vi "故障告警分析.vi"(8 "告警代码":u16, 9 "故障代码":u16, 10 "运行步序":u16, 11 "参数":string) -> (1 "报警簇":T1, 2 "报警内容":T2, 3 "简易报警状态":cluster{"故障状态":string, "报警状态":string}, 5 "sysid":i32)   [LabVIEW 2016, in "斯坦道氨氮.lvlib"]
panel:
  in  "氨氮报警":string[][](array[string])
  # "1、注射泵水样阀口堵塞；\n2、注射泵阀过载或丝杆无动作。"
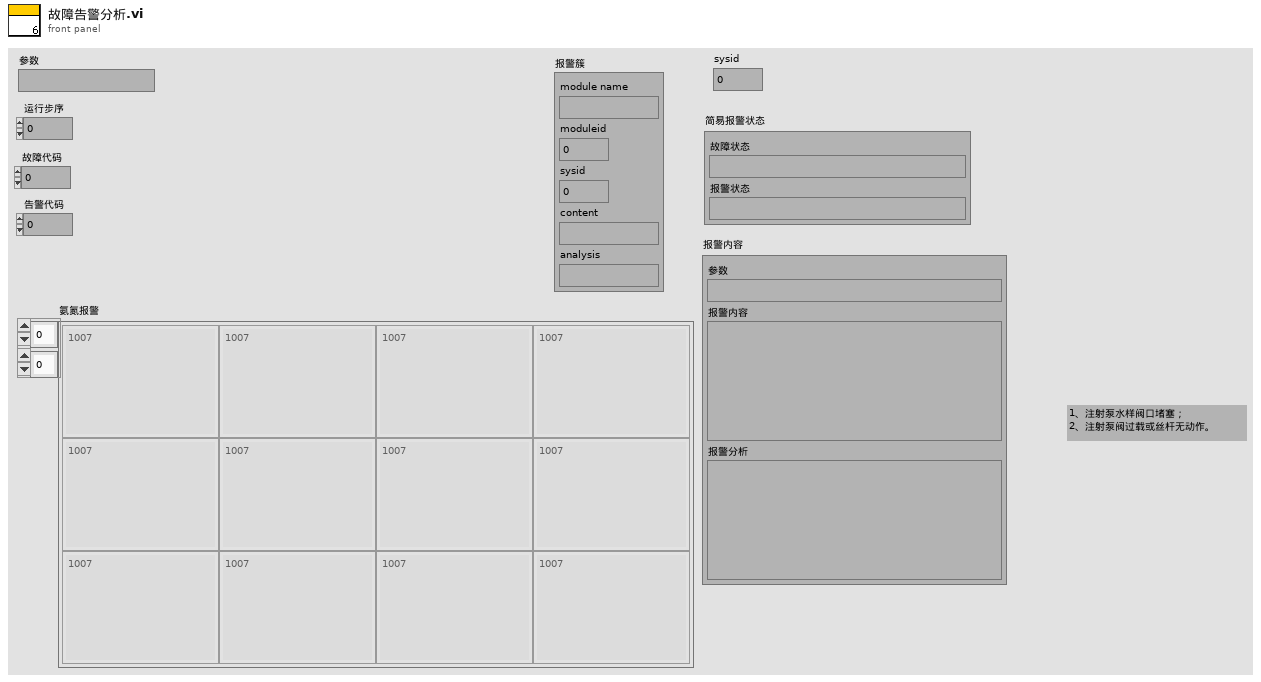
[diagram p1: front panel]
types:
  T1 = cluster{"module name":string, "moduleid":i32, "sysid":i32, "content":string, "analysis":string}
  T2 = cluster{"参数":string, "报警内容":string, "报警分析":string}
  T3 = cluster{"modid":i32, "sysid":i32, "content":string, "故障详情":string}
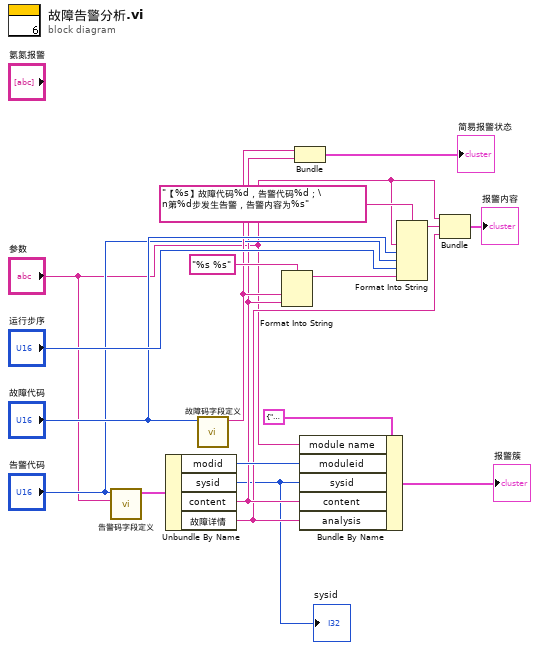
[diagram p0: block diagram]
diagram:
  n1 = call "告警码字段定义.vi"("模块名称"="参数", "告警代码"="告警代码") -> ("报警"=w6:T3)  [unwired: 9 in]
  n2 = Unbundle By Name(w6) -> ("modid"=w5:i32, "sysid"=w1:i32, "content"=w4:string, "故障详情"=w3:string)
  "sysid" <- w1
  n3 = call "故障码字段定义.vi"("故障代码"="故障代码") -> ("字符串"=w12:string)  [unwired: 10 in]
  n4 = Format Into String(format string="%s %s" ("格式字符串"), w12, w4) -> (resulting string=w8:string)  [unwired: 2 in, 1 out]
  n5 = Bundle("字符串"=w12, "content"=w4) -> (→"简易报警状态":cluster{"字符串":string, "content":string})  [unwired: 1 in]
  n6 = Bundle By Name(cluster=T1 {"module name"="", "moduleid"=0, "sysid"=0, "content"="", "analysis"=""} ("簇"), "module name"="参数", "moduleid"=w5, "sysid"=w1, "content"=w4, "analysis"=w3) -> (→"报警簇":T1)
  n7 = Format Into String(format string="【%s】故障代码%d，告警代码%d；\n第%d步发生告警，告警内容为%s" ("格式字符串"), "参数", "故障代码", "告警代码", "运行步序", w8) -> (resulting string=w9:string)  [unwired: 2 in, 1 out]
  n8 = Bundle("参数"="参数", w9, "故障详情"=w3) -> (→"报警内容":cluster{"参数":string, string, "故障详情":string})  [unwired: 1 in]
